vi "GitHub API_List Releases.vi"() -> ()   [LabVIEW 2013]
uses:
  <vilib>/httpClient/LabVIEWHTTPClient.lvlib
  <vilib>/addons/_JKI.lib/Serialization/JSON/JKI JSON Serialization.lvlib
panel:
  out "Releases":T1(array[cluster])
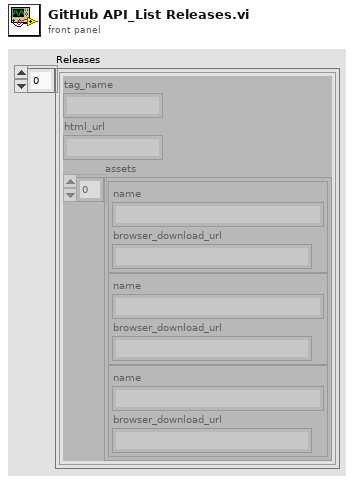
[diagram p1: front panel]
types:
  T1 = cluster{"tag_name":string, "html_url":string, "assets":cluster{"name":string, "browser_download_url":string}[]}[]
  T2 = typedef "LabVIEWHTTPClient.lvlib/ClientHandle.ctl" = refnum<k1>
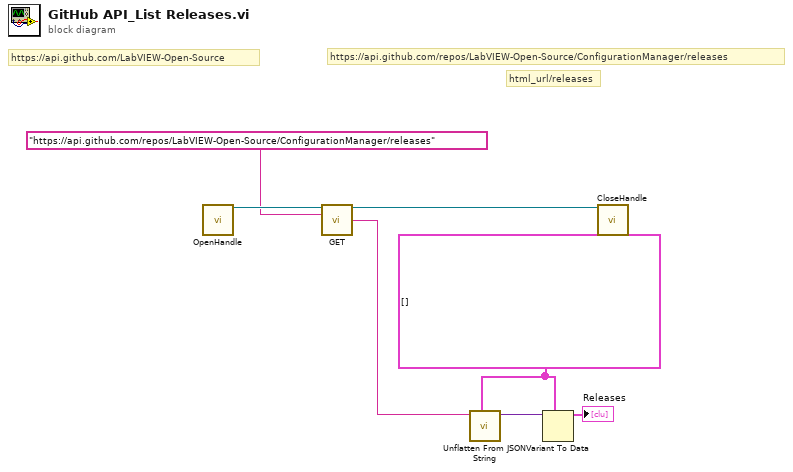
[diagram p0: block diagram]
diagram:
  w2 = T1 []
  # "https://api.github.com/repos/LabVIEW-Open-Source/ConfigurationManager/releases"
  # "html_url/releases"
  # "https://api.github.com/LabVIEW-Open-Source"
  n1 = call <vilib>:"OpenHandle.vi"() -> ("client handle out"=w7:T2)  [unwired: 14 in, 1 out]
  n2 = call <vilib>:"GET.vi"("client handle"=w7, "url"="https://api.github.com/repos/LabVIEW-Open-Source/ConfigurationManager/releases") -> ("client handle out"=w5:T2, "body"=w4:string)  [unwired: 10 in, 2 out]
  n3 = call <vilib>:"Unflatten From JSON String.vi"("Type and Defaults"=w2, "JSON String"=w4) -> ("Variant"=w3:variant)  [unwired: 8 in, 1 out]
  n4 = Variant To Data(type=w2, Variant=w3) -> (data=→"Releases":T1)  [unwired: 1 in, 1 out]
  n5 = call <vilib>:"CloseHandle.vi"("client handle"=w5) -> ()  [unwired: 14 in, 1 out]
